vi "Encode UTF-8 Path.vi"(5 "Prepend BOM (F)":bool, 7 "Output Encoding (UTF-16LE)":T1=enum."UTF-16LE", 9 "error in (no error)":errorcluster, 10 "UTF-8 Path":refnum<class "UTF-8 Path.lvclass">) -> (1 "error out":errorcluster, 2 "Encoded Path":string)   [LabVIEW 2020, in "G-Unicode.lvlib" / "UTF-8 Path.lvclass"]
doc: "Encodes the input <b>UTF-8 Path</b> using the specified <b>Output Encoding</b>."
uses:
  Unicode/Controls/String Encoding.ctl
  UTF-8 String/UTF-8 String.lvclass/UTF-8 String.ctl
  Private/Conversion/Text to UTF-8.vi
  Private/Conversion/Polymorphic VIs/Text to UTF-8 (LabVIEW String).vi
  Private/Conversion/Encoded UTF-8 String to Encoded UTF-16LE String.vi
  Private/Conversion/UTF-8 to Text.vi
  Private/Conversion/Polymorphic VIs/UTF-8 to Text (LabVIEW String).vi
  Private/Conversion/Encoded UTF-16LE String to Encoded UTF-8 String.vi
  Unicode/Prepend BOM.vi
  Unicode/SubVIs/Byte Order Marks.vi
  Unicode/Detect BOM.vi
  Unicode/Detect String Encoding.vi
  UTF-8 Path.lvclass
  G-Unicode.lvlib
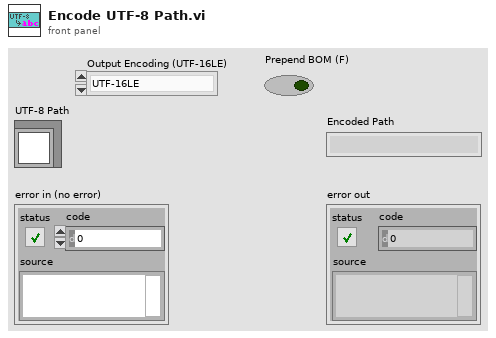
[diagram p1: front panel]
types:
  T1 = typedef "G-Unicode.lvlib/String Encoding.ctl" = enum16{"ANSI", "UTF-8", "UTF-16LE", "UTF-16BE", "Unknown"}
  T2 = typedef "G-Unicode.lvlib/Encoded UTF-8 Path.ctl" = path
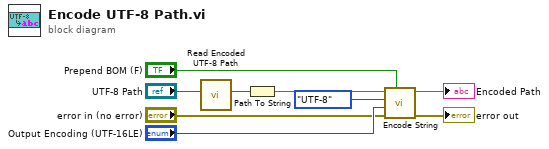
[diagram p0: block diagram]
diagram:
  n1 = call "Read Encoded UTF-8 Path.vi"("UTF-8 Path"="UTF-8 Path") -> ("Encoded UTF-8 Path"=w8:T2)  [unwired: 10 in]
  n2 = Path To String(path=w8) -> (string=w1:string)
  n3 = call "Encode String.vi"("Prepend BOM (F)"="Prepend BOM (F)", "error in"="error in (no error)", "Output Encoding (UTF-16LE)"="Output Encoding (UTF-16LE)", "Input Encoding (ANSI)"=String_Encoding."UTF-8", "String in"=w1) -> ("error out"=→"error out":errorcluster, "String out"=→"Encoded Path":string)  [unwired: 5 in]
